vi "SQLiteError.vi"(4 "ConfigCommand":T1, 5 "error in (no error)":errorcluster, 7 "ErrorData":string[](array[string]), 8 "ErrorNumber":string) -> (0 "error out":errorcluster, 2 "All Errors":string[][](array[string]), 3 "#Errors":i32)   [LabVIEW 2018]
doc: "*-----------------------------------------------------\n* Author: SWatts\n*\n* VI Description: Configuration dialog\n* \n*\n* Error handling: All errors passed out\n*\n* Pre-condition: \n*\n* Post-condition: None\n*\n* Revision History:\n*\n* Rev Date Author Description \n* 01 30/04/2014 SWatts First issue\n*\n*-----------------------------------------------------"
uses:
  ErrordBCommand.ctl
  Database/SystemdBCommands.ctl
panel:
  # "Output"
  # "Input"
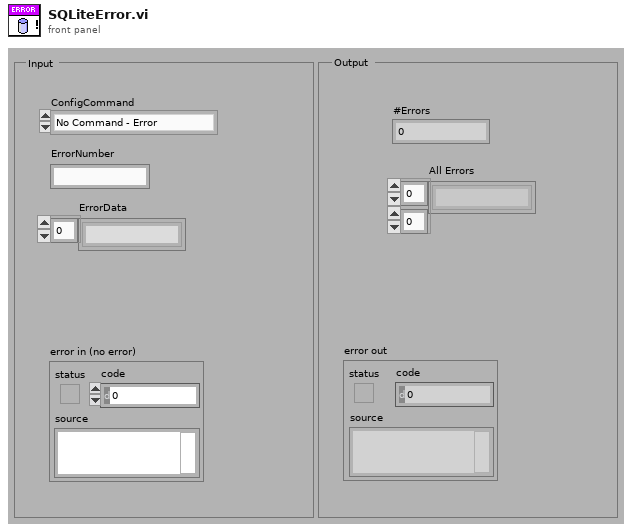
[diagram p1: front panel]
types:
  T1 = typedef "ErrordBCommand.ctl" = enum16{"No Command - Error", "Get All Errors", "Get #Errors", "Clear Error Log", "Insert New Error", "Update Existing Error"}
  T2 = typedef "SystemdBCommands.ctl" = enum16{"No Command - Error", "Set Filepath", "Connect dB", "Disconnect dB", "Start Transaction", "Commit", "Rollback", "Describe Table", "Select All From Table", "Fetch Query", "Count Records In Table", "Get User Information", "Get System Config", "Insert New System Config", "UPDATE User Info", "Insert New User", "Get Versions", "Update Key", "Set Version to Default", "Get Default Version", "INSERT Error", "UPDATE Error", "DELETE Errors", "Get All Errors", "Get #Errors for Error"}
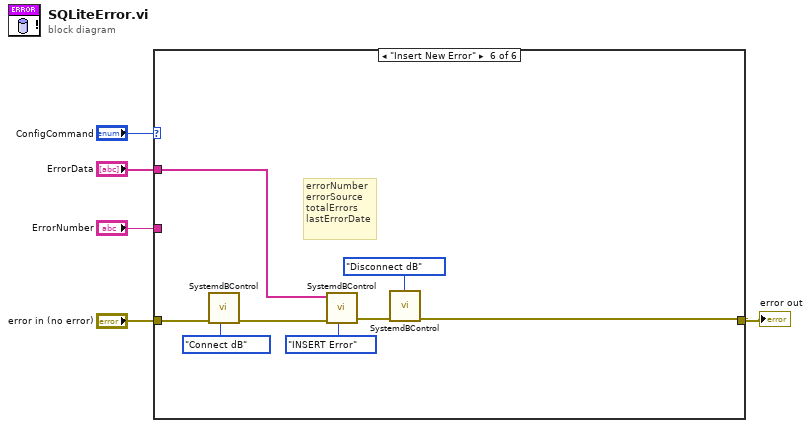
[diagram p0: block diagram]
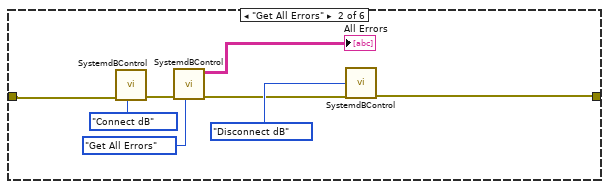
[diagram p3: hidden frame]
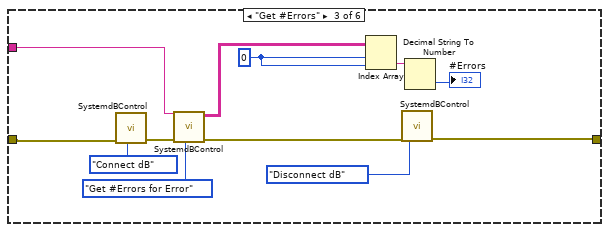
[diagram p4: hidden frame]
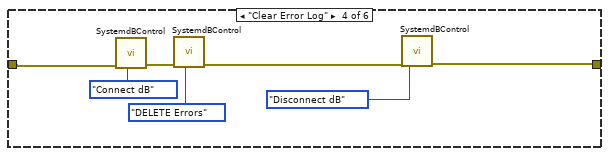
[diagram p5: hidden frame]
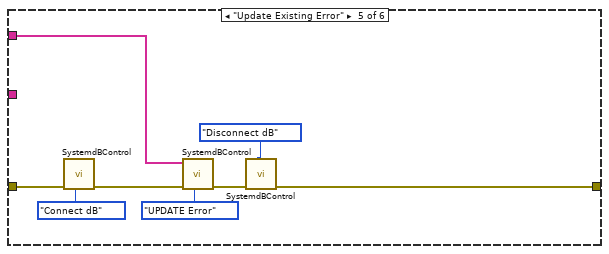
[diagram p6: hidden frame]
diagram:
  n1 = case shown="\"Insert New Error\"" "ConfigCommand" {
    tunnel: "error in (no error)" -> [w6 w12 w24 w31 w38 w45]
    tunnel: [w6 w11 w23 w30 w37 w44] -> w3
    tunnel: "ErrorNumber" -> [_ _ w19 _ _ _]
    tunnel: "ErrorData" -> [_ _ _ _ w35 w42]
    frame "No Command - Error", Default {
    }
    frame "Get All Errors" {
      n2 = call "SystemdBControl.vi"("Command"=SystemdBCommands."Connect dB", "error in (no error)"=w12) -> ("error out"=w10:errorcluster)  [unwired: 5 in, 2 out]
      n3 = call "SystemdBControl.vi"("Command"=SystemdBCommands."Get All Errors", "error in (no error)"=w10) -> ("error out"=w8:errorcluster, "Data Out"=→"All Errors":string[][])  [unwired: 5 in, 1 out]
      n4 = call "SystemdBControl.vi"("Command"=SystemdBCommands."Disconnect dB", "error in (no error)"=w8) -> ("error out"=w11:errorcluster)  [unwired: 5 in, 2 out]
    }
    frame "Get #Errors" {
      w17 = 0 ("index (row)")
      n5 = call "SystemdBControl.vi"("Command"=SystemdBCommands."Connect dB", "error in (no error)"=w24) -> ("error out"=w22:errorcluster)  [unwired: 5 in, 2 out]
      n6 = call "SystemdBControl.vi"("Command"=SystemdBCommands."Get #Errors for Error", "error in (no error)"=w22, "Data In"=w19) -> ("error out"=w20:errorcluster, "Data Out"=w18:string[][])  [unwired: 4 in, 1 out]
      n7 = Index Array(array=w18, index (row)=w17, index (col)=w17) -> (element=w16:string)
      n8 = call "SystemdBControl.vi"("Command"=SystemdBCommands."Disconnect dB", "error in (no error)"=w20) -> ("error out"=w23:errorcluster)  [unwired: 5 in, 2 out]
      n9 = Decimal String To Number(string=w16) -> (number=→"#Errors":i32)  [unwired: 2 in, 1 out]
    }
    frame "Clear Error Log" {
      n10 = call "SystemdBControl.vi"("Command"=SystemdBCommands."Connect dB", "error in (no error)"=w31) -> ("error out"=w29:errorcluster)  [unwired: 5 in, 2 out]
      n11 = call "SystemdBControl.vi"("Command"=SystemdBCommands."DELETE Errors", "error in (no error)"=w29) -> ("error out"=w27:errorcluster)  [unwired: 5 in, 2 out]
      n12 = call "SystemdBControl.vi"("Command"=SystemdBCommands."Disconnect dB", "error in (no error)"=w27) -> ("error out"=w30:errorcluster)  [unwired: 5 in, 2 out]
    }
    frame "Update Existing Error" {
      n13 = call "SystemdBControl.vi"("Command"=SystemdBCommands."Connect dB", "error in (no error)"=w38) -> ("error out"=w34:errorcluster)  [unwired: 5 in, 2 out]
      n14 = call "SystemdBControl.vi"("Command"=SystemdBCommands."UPDATE Error", "error in (no error)"=w34, "Data In"=w35) -> ("error out"=w39:errorcluster)  [unwired: 4 in, 2 out]
      n15 = call "SystemdBControl.vi"("Command"=SystemdBCommands."Disconnect dB", "error in (no error)"=w39) -> ("error out"=w37:errorcluster)  [unwired: 5 in, 2 out]
    }
    frame "Insert New Error" {
      # "errorNumber\nerrorSource\ntotalErrors\nlastErrorDate"
      n16 = call "SystemdBControl.vi"("Command"=SystemdBCommands."Connect dB", "error in (no error)"=w45) -> ("error out"=w48:errorcluster)  [unwired: 5 in, 2 out]
      n17 = call "SystemdBControl.vi"("Command"=SystemdBCommands."INSERT Error", "error in (no error)"=w48, "Data In"=w42) -> ("error out"=w46:errorcluster)  [unwired: 4 in, 2 out]
      n18 = call "SystemdBControl.vi"("Command"=SystemdBCommands."Disconnect dB", "error in (no error)"=w46) -> ("error out"=w44:errorcluster)  [unwired: 5 in, 2 out]
    }
  }
  "error out" <- w3
